vi "Start Call to results window.vi"(8 "Find Broadcast?":bool, 9 "Request VI Callers":refnum<vi>[](array[refnum]), 10 "Event":refnum<vi>, 11 "Theme":bool) -> ()   [LabVIEW 2019, in "Panther Dashboard.lvlib"]
uses:
  Panther Dashboard.lvlib
  Show Caller Items Dialog.vi
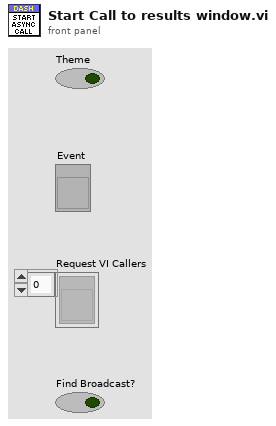
[diagram p1: front panel]
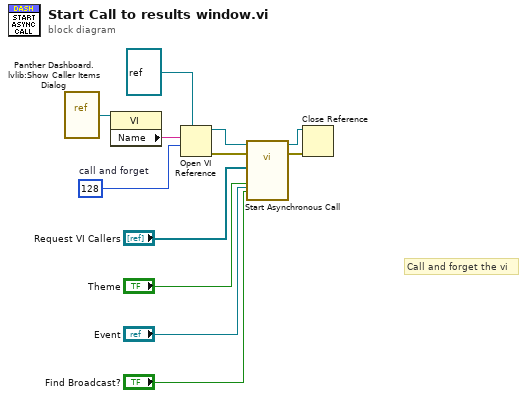
[diagram p0: block diagram]
diagram:
  w9 = 128  # call and forget
  # "Call and forget the vi"
  n1 = vi-ref "Panther Dashboard.lvlib:Show Caller Items Dialog.vi"() -> (w6:refnum<vi>)
  n2 = property class="VI"(reference=w6) -> ("Name"=w7:string)  [unwired: 1 in, 2 out]
  n3 = Open VI Reference(type specifier VI Refnum (for type only)=refnum<vi> refnum, vi path=w7, options=w9) -> (vi reference=w5:refnum<vi>, error out=w11:errorcluster)  [unwired: 3 in]
  n4 = call-by-ref "Start Asynchronous Call"(reference=w5, error in=w11, "Event"="Event", "Find Broadcast?"="Find Broadcast?", "Theme"="Theme", "Request VI Callers"="Request VI Callers") -> (reference out=w8:refnum<vi>, error out=w12:errorcluster)  [unwired: 8 in]
  n5 = Close Reference(reference=w8, error in (no error)=w12) -> ()  [unwired: 1 out]
